vi "Add PID Parameter Row.vi"(8 "error in (no error)":errorcluster, 11 "MulticolumnListbox in":refnum<vi>) -> (0 "error out":errorcluster)   [LabVIEW 2019, in "Control Addon Shared.lvlib"]
uses:
  Control Addon Shared.lvlib
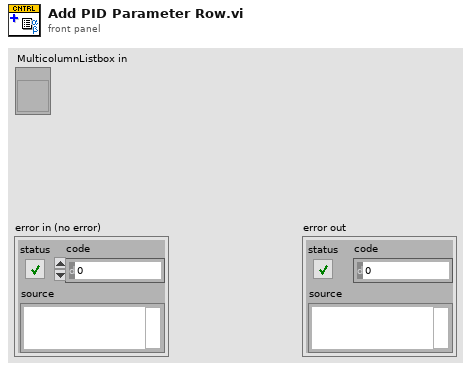
[diagram p1: front panel]
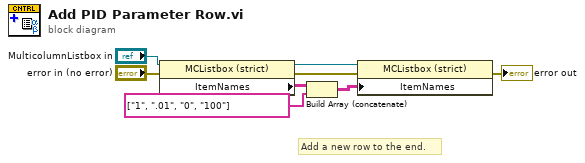
[diagram p0: block diagram]
diagram:
  # "Add a new row to the end."
  n1 = property class="MCListbox (strict)"(reference="MulticolumnListbox in", error in="error in (no error)") -> (reference out=w4:refnum<vi>, error out=w2:errorcluster, "ItemNames"=w5:string[][])
  n2 = Build Array (concatenate)(w5, string[] ["1", ".01", "0", "100"]) -> (w7:string[][])
  n3 = property class="MCListbox (strict)"(reference=w4, error in=w2, "ItemNames"=w7) -> (error out=→"error out":errorcluster)  [unwired: 1 out]
